vi "WriteLogFileToDisk.vi"(7 "Log File path":path, 8 "error in (no error)":errorcluster, 11 "Message":T1) -> (0 "error out":errorcluster)   [LabVIEW 2013, in "ErrorMessage.lvclass"]
uses:
  001 - MAIN/Class/Messages/ErrorMessage/ErrorMessage.lvclass
  030 - EVENTS/03 - ToMessageHandlerProcess/ToMessageHandlerEvent.ctl
  030 - EVENTS/03 - ToMessageHandlerProcess/enumMessageCriticity.ctl
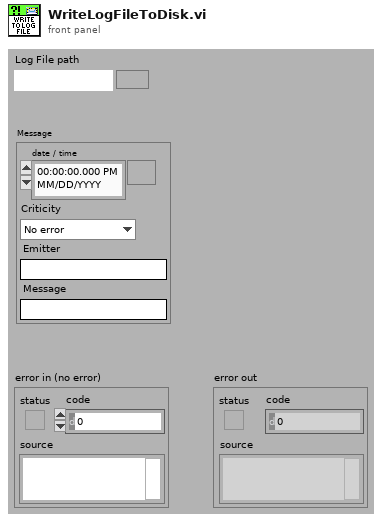
[diagram p1: front panel]
types:
  T1 = typedef "ToMessageHandlerEvent.ctl" = cluster{"date / time":timestamp, "Criticity":T2, "Emitter":string, "Message":string}
  T2 = typedef "enumMessageCriticity.ctl" = enum16{"No error", "Info", "Warning", "Error", "Fatal error"}
  T3 = enum16{"open", "replace", "create", "open or create", "replace or create", "replace or create with confirmation"}
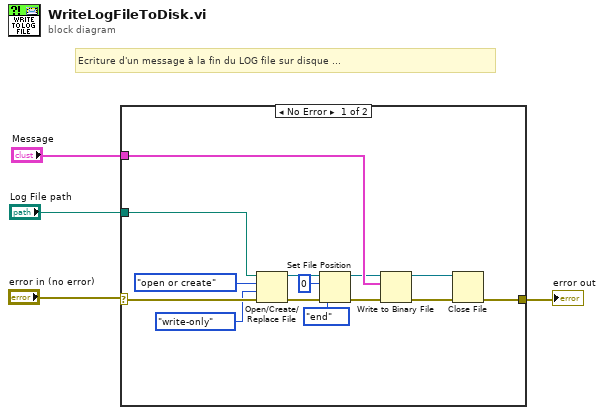
[diagram p0: block diagram]
diagram:
  # "Ecriture d'un message à la fin du LOG file sur disque ..."
  n1 = case shown="No Error" "error in (no error)" {
    selector: "error in (no error)" -> [w18 w19]
    tunnel: [w11 w19] -> w3
    tunnel: "Log File path" -> [w17 _]
    tunnel: "Message" -> [w14 _]
    frame No Error {
      n2 = Open/Create/Replace File(file path (use dialog)=w17, error in=w18, operation (0:open)=T3."open or create", access (0:read/write)=enum16{"read/write", "read-only", "write-only"}."write-only") -> (refnum out=w10:refnum<file>, error out=w8:errorcluster)  [unwired: 2 in, 1 out]
      n3 = Set File Position(offset (in bytes) (0)=i64 0, refnum=w10, from (0:start)=enum16{"start", "end", "current"}."end", error in=w8) -> (refnum out=w9:refnum<file>, error out=w7:errorcluster)
      n4 = Write to Binary File(file (use dialog)=w9, data=w14, error in=w7) -> (refnum out=w12:refnum<file>, error out=w13:errorcluster)  [unwired: 3 in, 1 out]
      n5 = Close File(refnum=w12, error in=w13) -> (error out=w11:errorcluster)  [unwired: 1 out]
    }
    frame Error {
    }
  }
  "error out" <- w3
